vi "RSZVB Get Virtual Transform Port Pair.vi"(0 "VISA session":refnum<visa-resource-name>, 1 "Parameter Type (Capacitance)":i32(ring) items=["Capacitance", "Inductance", "Resistance"], 2 "Circuit Model (Serial Touchstone (.s2p) data, shunt L)":i32(ring)=1 items=["Serial Touchstone (.s2p) data, shunt L"=1, "Serial Touchstone (.s2p) data, shunt C"=2, "Shunt L, serial Touchstone (.s2p) data"=3, "Shunt C, serial Touchstone (.s2p) data"=4, "Serial Cs, shunt L"=5, "Serial Ls, shunt C"=6, "Serial Cs, shunt C"=7, "Serial Ls, shunt L"=8, "Shunt L, serial Cs"=9, "Shunt C, serial Ls"=10, "Shunt C, serial Cs"=11, "Shunt L, serial Ls"=12], 5 "Channel (1)":i32=1, 7 "Function Type (Deembedding)":i32(ring) items=["Deembedding", "Embedding"], 9 "Port Pair (1)":i32=1, 11 "error in (no error)":errorcluster {"code" format="%.0x"}, 12 "Parameter Number (1)":i32=1) -> (4 "dup VISA session":refnum<visa-resource-name>, 6 "Value":dbl format="%^.3e", 15 "error out":errorcluster {"code" format="%.0x"})   [LabVIEW 2011]
doc: "This VI queries the capacitance, inductance or resistance values C1, C2, C3, L1, L2, L3 or R1, R2, R3 in the different circuit models for port pair deembedding/embedding.\n\nRemote-control command(s):\nCALCulate<Ch>:TRANsform:VNETworks:PPAir:DEEMbedding<List_idx>:PARameters:C<no>? STSC | SCST | CSSL | LSSC | CSSC | SLCS | SCLS | SCCS,<numeric_value>\nCALCulate<Ch>:TRANsform:VNETworks:PPAir:DEEMbedding<List_idx>:PARameters:L<no>? STSL | SLST | CSSL | LSSC | LSSL | SLCS | SCLS | SLLS,<numeric_value>\nCALCulate<Ch>:TRANsform:VNETworks:PPAir:DEEMbedding<List_idx>:PARameters:R<no>? STSL | STSC | SLST | SCST | CSSL | LSSC | CSSC | LSSL | SLCS | SCLS | SCCS | SLLS,<numeric_value>\nCALCulate<Ch>:TRANsform:VNETworks:PPAir:EMBedding<List_idx>:PARameters:C<no>? STSC | SCST | CSSL | LSSC | CSSC | SLCS | SCLS | SCCS,<numeric_value>\nCALCulate<Ch>:TRANsform:VNETworks:PPAir:EMBedding<List_idx>:PARameters:L<no>? STSL | SLST | CSSL | LSSC | LSSL | SLCS | SCLS | SLLS,<numeric_value>\nCALCulate<Ch>:TRANsform:VNETworks:PPAir:EMBedding<List_idx>:PARameters:R<no>? STSL | STSC | SLST | SCST | CSSL | LSSC | CSSC | LSSL | SLCS | SCLS | SCCS | SLLS,<numeric_value>"
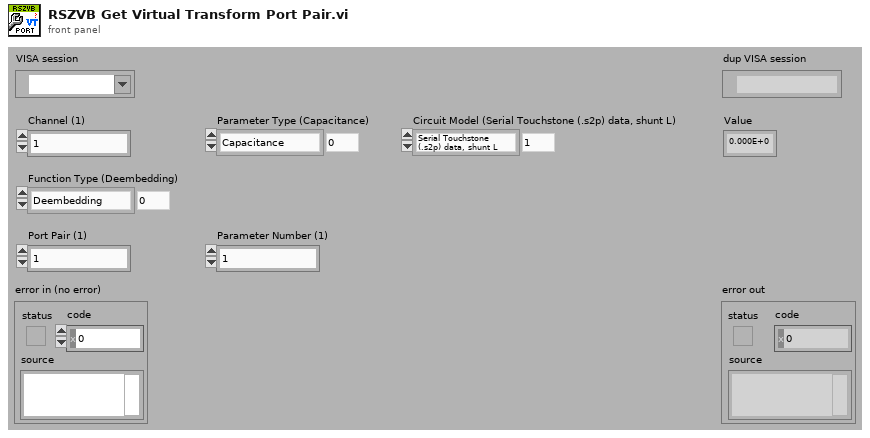
[diagram p1: front panel]
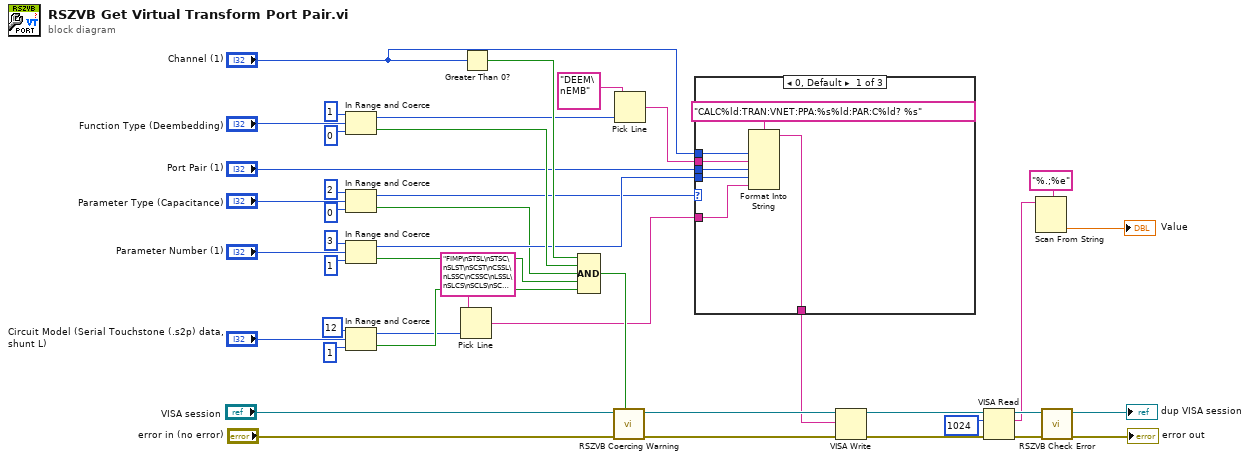
[diagram p0: block diagram]
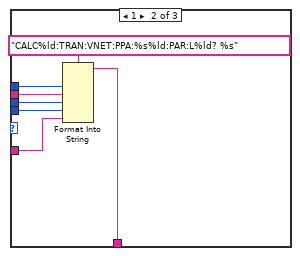
[diagram p2: hidden frame]
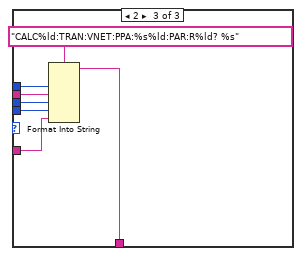
[diagram p3: hidden frame]
diagram:
  n1 = In Range and Coerce(upper limit=1 ("lower limit"), x="Function Type (Deembedding)", lower limit=0) -> (coerced(x)=w35:i32, In Range?=w37:bool)
  n2 = In Range and Coerce(upper limit=2 ("lower limit"), x="Parameter Type (Capacitance)", lower limit=0) -> (coerced(x)=w23:i32, In Range?=w26:bool)
  n3 = In Range and Coerce(upper limit=3 ("lower limit"), x="Parameter Number (1)", lower limit=1) -> (coerced(x)=w27:i32, In Range?=w25:bool)
  n4 = In Range and Coerce(upper limit=12 ("lower limit"), x="Circuit Model (Serial Touchstone (.s2p) data, shunt L)", lower limit=1) -> (coerced(x)=w7:i32, In Range?=w24:bool)
  n5 = Pick Line(multi-line string="FIMP\nSTSL\nSTSC\nSLST\nSCST\nCSSL\nLSSC\nCSSC\nLSSL\nSLCS\nSCLS\nSCCS\nSLLS", line index=w7) -> (output string=w6:string)  [unwired: 1 in]
  n6 = Greater Than 0?(x="Channel (1)") -> (x > 0?=w39:bool)
  n7 = Compound Arithmetic op=AND(w39, w37, w26, w25, w24) -> (w38:bool)
  n8 = call "RSZVB Coercing Warning.vi"("In Range?"=w38, "error in (no error)"="error in (no error)", "VISA session"="VISA session") -> ("error out"=w42:errorcluster, "dup VISA session"=w43:refnum<visa-resource-name>)  [unwired: 7 in]
  n9 = Pick Line(multi-line string="DEEM\nEMB", line index=w35) -> (output string=w34:string)  [unwired: 1 in]
  n10 = case shown="0, Default" w23 {
    tunnel: w34 -> [w49 w56 w63]
    tunnel: w27 -> [w48 w55 w62]
    tunnel: [w47 w54 w61] -> w22
    tunnel: "Channel (1)" -> [w46 w51 w58]
    tunnel: "Port Pair (1)" -> [w45 w52 w59]
    tunnel: w6 -> [w44 w53 w60]
    frame 0, Default {
      n11 = Format Into String(format string="CALC%ld:TRAN:VNET:PPA:%s%ld:PAR:C%ld? %s", w46, w49, w45, w48, w44) -> (resulting string=w47:string)  [unwired: 2 in, 1 out]
    }
    frame 1 {
      n12 = Format Into String(format string="CALC%ld:TRAN:VNET:PPA:%s%ld:PAR:L%ld? %s", w51, w56, w52, w55, w53) -> (resulting string=w54:string)  [unwired: 2 in, 1 out]
    }
    frame 2 {
      n13 = Format Into String(format string="CALC%ld:TRAN:VNET:PPA:%s%ld:PAR:R%ld? %s", w58, w63, w59, w62, w60) -> (resulting string=w61:string)  [unwired: 2 in, 1 out]
    }
  }
  n14 = VISA Write(VISA resource name=w43, write buffer=w22, error in (no error)=w42) -> (VISA resource name out=w15:refnum<visa-resource-name>, error out=w16:errorcluster)  [unwired: 1 out]
  n15 = VISA Read(VISA resource name=w15, byte count=u32 1024 ("byte count (0)"), error in (no error)=w16) -> (VISA resource name out=w20:refnum<visa-resource-name>, read buffer=w17:string, error out=w19:errorcluster)  [unwired: 1 out]
  n16 = Scan From String(format string="%.;%e", input string=w17) -> (output 1=→"Value":dbl)  [unwired: 3 in, 3 out]
  n17 = call "RSZVB Check Error.vi"("error in (no error)"=w19, "VISA session"=w20) -> ("error out"=→"error out":errorcluster, "dup VISA session"=→"dup VISA session":refnum<visa-resource-name>)  [unwired: 8 in]
